vi "Async Heartbeat.vi"(10 "Main VI":string, 11 "Ethernet out":refnum<class "ENET_BS120x.lvclass">) -> ()   [LabVIEW 2021, in "BS120x Driver.lvlib" / "ENET_BS120x.lvclass"]
uses:
  ENET_BS120x.lvclass
  ENET_BS120x.lvclass/ENET_BS120x.ctl
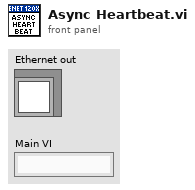
[diagram p1: front panel]
types:
  T1 = enum32{"Bad", "Idle", "Run top level", "Running"}
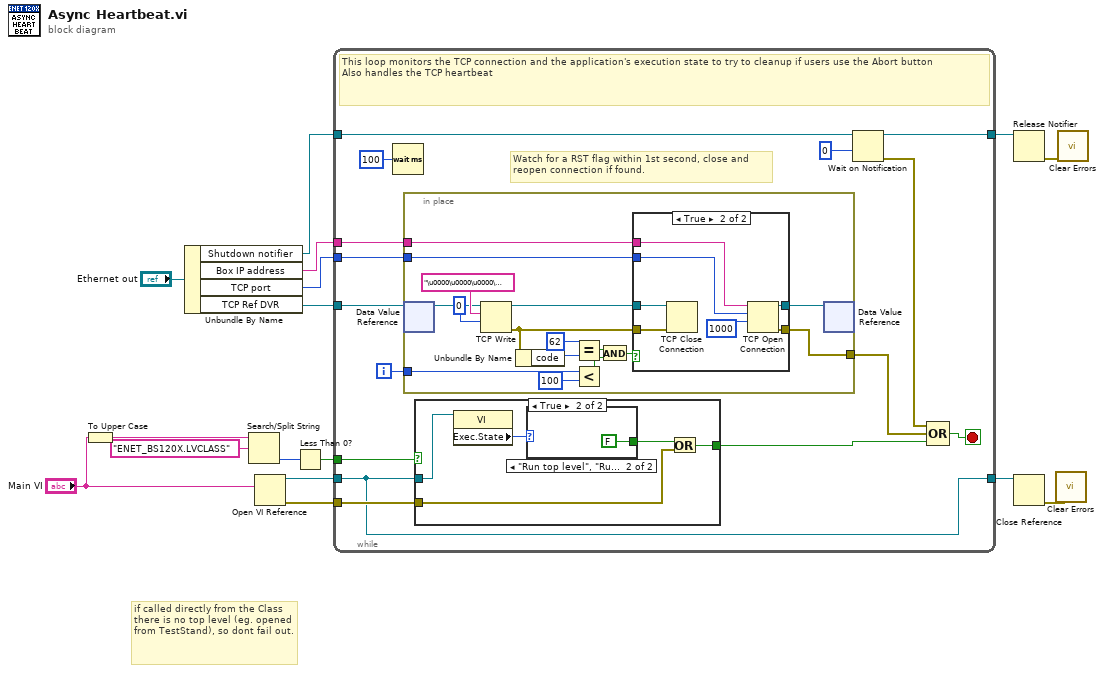
[diagram p0: block diagram]
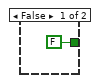
[diagram p2: hidden frame]
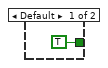
[diagram p3: hidden frame]
diagram:
  # "if called directly from the Class there is no top level (eg. opened from TestStand), so dont fail out."
  n1 = To Upper Case(1:"Main VI") -> (0:w5:string)
  n2 = Unbundle By Name("Ethernet out") -> ("Shutdown notifier"=w8:refnum<notifier>, "Box IP address"=w10:string, "TCP port"=w9:u16, "TCP Ref DVR"=w11:refnum<data-value>)
  n3 = Search/Split String(string=w5, search string/char (-)="ENET_BS120X.LVCLASS") -> (offset of match=w4:i32)  [unwired: 1 in, 2 out]
  n4 = Open VI Reference(vi path="Main VI") -> (vi reference=w15:refnum<vi>, error out=w14:errorcluster)  [unwired: 5 in]
  n5 = Less Than 0?(x=w4) -> (x < 0?=w3:bool)
  n6 = while {
    tunnel: w15 -> [w17]
    tunnel: w14 -> [w20]
    tunnel: [w17] -> w13
    tunnel: w11 -> [w24]
    tunnel: w10 -> [w21]
    tunnel: w9 -> [w22]
    tunnel: w8 -> [w28]
    tunnel: [w27] -> w16
    tunnel: w3 -> [w18]
    i -> [w23]
    stop <- w31 stop-if-true
    # "Watch for a RST flag within 1st second, close and\nreopen connection if found."
    # "This loop monitors the TCP connection and the application's execution state to try to cleanup if users use the Abort button\nAlso handles the TCP heartbeat"
    n7 = Wait (ms)(milliseconds to wait=u32 100) -> ()  [unwired: 1 out]
    n8 = in-place {
      in-place-border: [w50] -> w25
      in-place-border: w23 -> [w41]
      in-place-border: w22 -> [w49]
      in-place-border: w21 -> [w48]
      n9 = in-place-dvr #1(w24) -> (w53:refnum<k5>)  [unwired: 1 out]
      n10 = TCP Write(connection ID=w53, data in="\u0000\u0000\u0000\u0001\u0001" ("concatenated string"), 9:0 ("timeout ms (25000)")) -> (connection ID out=w52:refnum<k5>, error out=w47:errorcluster)  [unwired: 1 in, 1 out]
      n11 = Unbundle By Name(w47) -> ("code"=w46:i32)
      n12 = Equal?(x=62, y=w46) -> (x = y?=w43:bool)
      n13 = Less?(x=w41, y=100) -> (x < y?=w42:bool)
      n14 = And(x=w43, y=w42) -> (x .and. y?=w44:bool)
      n15 = case shown="True" w44 {
        tunnel: w47 -> [w56 w64]
        tunnel: w52 -> [w57 w63]
        tunnel: [w56 w62] -> w50
        tunnel: [w57 w61] -> w51
        tunnel: w49 -> [_ w59]
        tunnel: w48 -> [_ w58]
        frame False {
        }
        frame True {
          n16 = TCP Close Connection(connection ID=w63, error in (no error)=w64) -> ()  [unwired: 1 in, 2 out]
          n17 = TCP Open Connection(address=w58, remote port or service name=w59, timeout ms (60000)=1000) -> (connection ID=w61:refnum<k5>, error out=w62:errorcluster)  [unwired: 2 in]
        }
      }
      n18 = in-place-dvr #1(w51) -> ()  [unwired: 2 out]
    }
    n19 = case shown="True" w18 {
      tunnel: w17 -> [_ w36]
      tunnel: w20 -> [_ w34]
      tunnel: [FALSE w33] -> w19
      frame False {
      }
      frame True {
        n20 = property class="VI"(reference=w36) -> ("Exec.State"=w37:T1)  [unwired: 1 in, 2 out]
        n21 = case shown="\"Run top level\", \"Running\"" w37 {
          tunnel: [TRUE FALSE] -> w35
          frame Default {
          }
          frame "Run top level", "Running" {
          }
        }
        n22 = Or(x=w35, y=w34) -> (x .or. y?=w33:bool)
      }
    }
    n23 = Wait on Notification(notifier=w28, timeout in ms (-1)=0) -> (notifier out=w27:refnum<notifier>, error out=w26:errorcluster)  [unwired: 2 in, 2 out]
    n24 = Compound Arithmetic op=OR(w26, w25, w19) -> (w31:bool)
  }
  n25 = Release Notifier(notifier=w16) -> (error out=w1:errorcluster)  [unwired: 2 in, 2 out]
  n26 = Close Reference(reference=w13) -> (error out=w2:errorcluster)  [unwired: 1 in]
  n27 = call <vilib>:"Clear Errors.vi"("error in (no error)"=w2) -> ()  [unwired: 5 in, 2 out]
  n28 = call <vilib>:"Clear Errors.vi"("error in (no error)"=w1) -> ()  [unwired: 5 in, 2 out]
